vi "3D Graph Properties - Torus.vi"() -> ()   [LabVIEW 2009]
doc: "Uses the CWGraph3D Active X control and the 3D Parametric Surface.vi to display a 3D parametric torus surface. Using the Basic Properties.vi, the plot style (8 style choices) and transparancy level (%) of the graph can be controlled.\n\nVIs Used:\n3D Parametric Surface.vi\nBasic Properties.vi"
uses:
  <vilib>/Platform/NI_3dgraph.lvlib
panel:
  in  "Numeric":i32
  in  "z matrix":dbl[][](array[numeric]) format="%.2f"
  in  "x matrix":dbl[][](array[numeric])
  in  "y matrix":dbl[][](array[numeric]) format="%.2f"
  out "Array":dbl[][](array[numeric])
  in  "Plot Style":i32(ring)=5 items=["cwLine"=1, "cwPoint"=2, "cwLinePoint"=3, "cwHiddenLine"=4, "cwSurface"=5, "cwSurfaceLine"=6, "cwSurfaceNormal"=7, "cwContourLine"=8, "cwSurfaceContour"=9]
  in  "Transparency (%)":dbl(knob)=1.3189706166826745 scale=0.0..100.0 scale format="%0.2f"
  in  "stop":bool
  in  "3D Graph":refnum<k7>(container)
  # "Instructions:\nSelect the desired plot style (8 choices) and transparancy level (%) and run the VI.  Control values may be changed while\nthe VI is running.  Additionally, the view of the 3D graph can be changed by positioning the mouse pointer over the graph,\nholding down the left mouse button, rotating the graph to the desired position, and releasing the left mouse button.  Press\nthe stop button to quit."
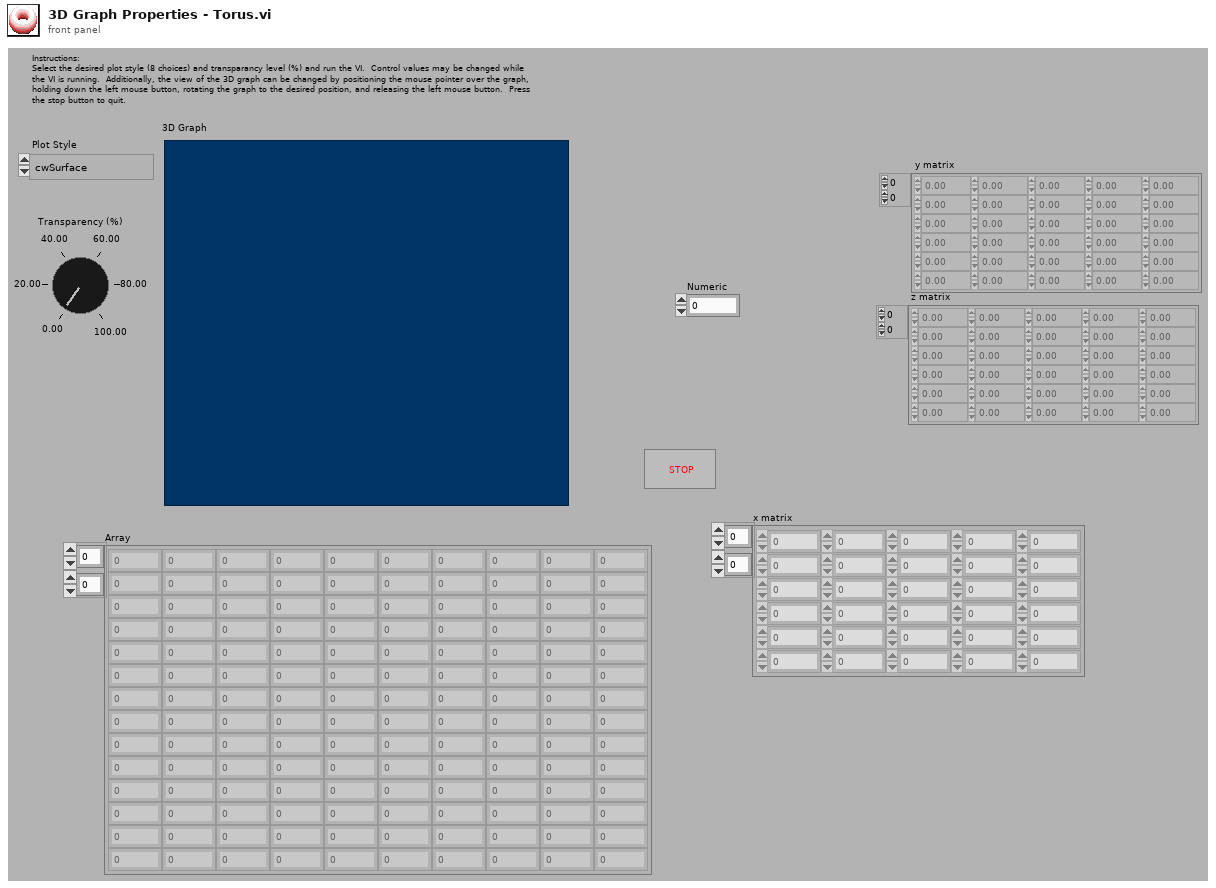
[diagram p1: front panel]
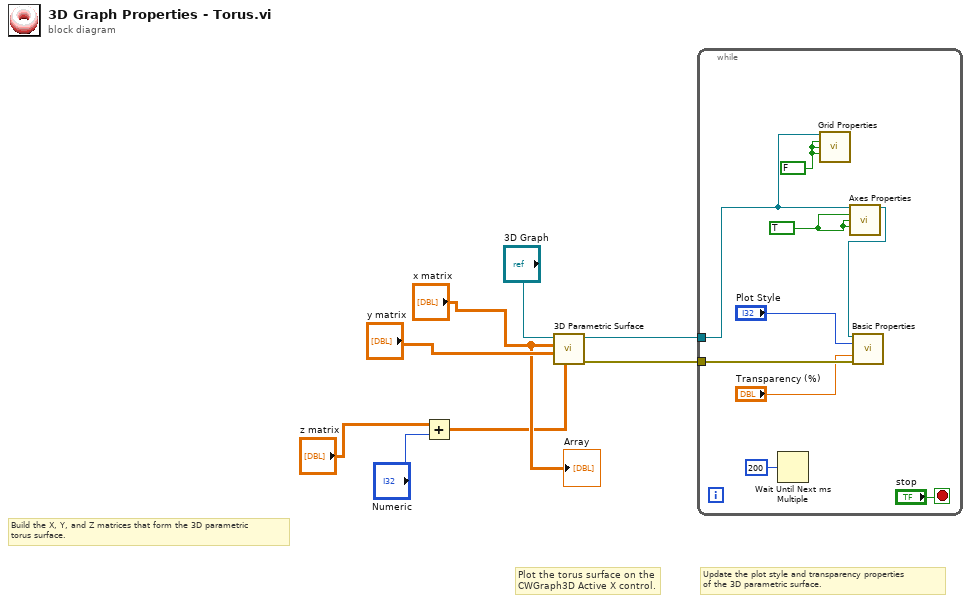
[diagram p0: block diagram]
diagram:
  # "Update the plot style and transparency properties\nof the 3D parametric surface."
  # "Plot the torus surface on the\nCWGraph3D Active X control."
  # "Build the X, Y, and Z matrices that form the 3D parametric\ntorus surface."
  n1 = Add(x="z matrix", y="Numeric") -> (x+y=w1:dbl[][])
  n2 = call <vilib>:"3D Parametric Surface.vi"("z matrix"=w1, "y matrix"="y matrix", "x matrix"="x matrix", "3D graph"="3D Graph") -> ("error out"=w6:errorcluster, "3D graph out"=w7:refnum<k7>)  [unwired: 6 in]
  n3 = while {
    tunnel: w6 -> [w17]
    tunnel: w7 -> [w10]
    stop <- "stop" stop-if-true
    w9 = FALSE ("auto scale x")
    w12 = TRUE ("auto scale x")
    n4 = Wait Until Next ms Multiple(millisecond multiple=u32 200) -> ()  [unwired: 1 out]
    n5 = call <vilib>:"Grid Properties.vi"("3D graph"=w10, "xy grid"=w9, "xz grid"=w9, "yz grid"=w9) -> ()  [unwired: 10 in, 2 out]
    n6 = call <vilib>:"Axes Properties.vi"("3D graph"=w10, "auto scale x"=w12, "auto scale y"=w12, "auto scale z"=w12) -> ("3D graph out"=w11:refnum<k7>)  [unwired: 10 in, 1 out]
    n7 = call <vilib>:"Basic Properties.vi"("3D graph"=w11, "plot style"="Plot Style", "transparency"="Transparency (%)", "error in (no error)"=w17) -> ()  [unwired: 10 in, 2 out]
  }
  "Array" <- "x matrix"
